vi "_Set PIC.vi"(1 "Count(uSec)":u8=20, 2 "Data":u32, 3 "Delay":u16) -> (0 "PIC Monitor":u32)   [LabVIEW 2018]
uses:
  <vilib>/eio/EIONode/EIONode.xnode
  <vilib>/rvi/DataTransferAndStorage/Container/XNode/niFpgaContainer.xnode
  <vilib>/rvi/eio/common/nirviEmuTemplateMethod_errors.vi
  <vilib>/rvi/Memory/Memory_Emulation/nirvimemoryFastEmulation.vi
  <vilib>/rvi/Memory/Memory_Emulation/nirvimemoryEmulation.vi
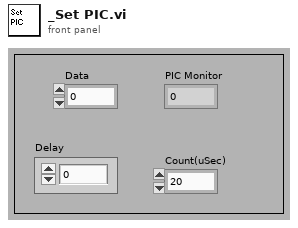
[diagram p1: front panel]
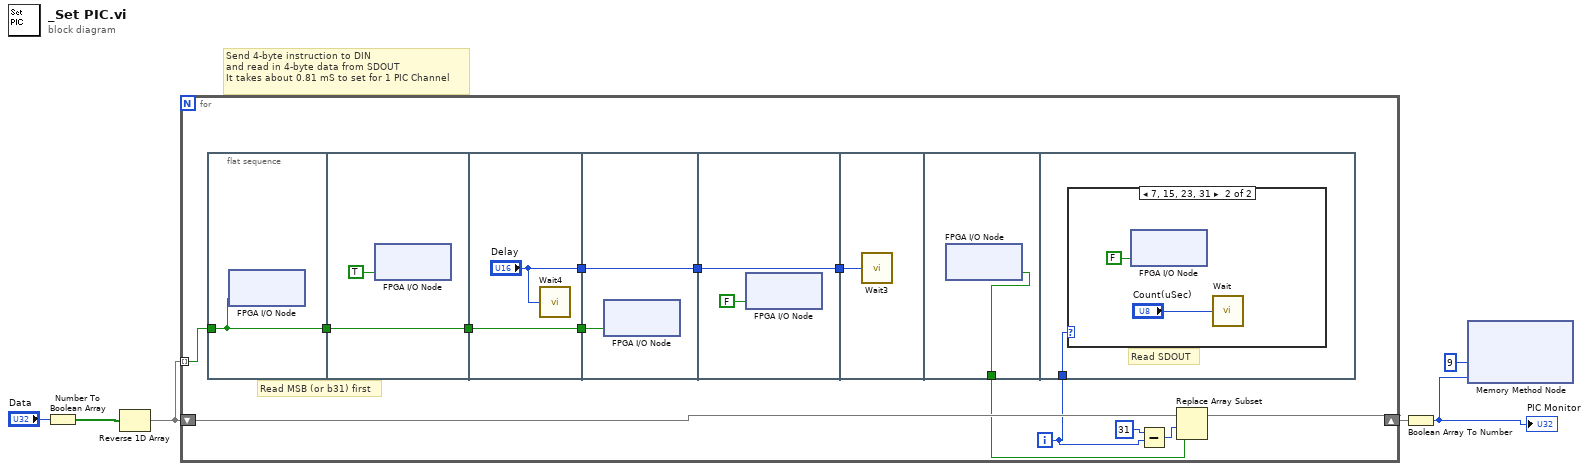
[diagram p0: block diagram]
diagram:
  # "Send 4-byte instruction to DIN\nand read in 4-byte data from SDOUT\nIt takes about 0.81 mS to set for 1 PIC Channel"
  n1 = Number To Boolean Array(number="Data") -> (Boolean array=w2:bool[])
  n2 = Reverse 1D Array(array=w2) -> (reversed array=w3:bool[])
  n3 = for {
    shift-right: [w18] -> w5
    shift-left: w3 -> [w19]
    tunnel: w3 -> [w15] mode=indexing
    i -> [w14]
    # "Read MSB (or b31) first"
    n4 = flat-sequence {
      tunnel: [w20] -> w11
      tunnel: w15 -> [w20]
      tunnel: w11 -> [w22]
      tunnel: [w22] -> w10
      tunnel: w10 -> [w24]
      tunnel: [w24] -> w13
      tunnel: ["Delay"] -> w12
      tunnel: w13 -> [w26]
      tunnel: [w25] -> w9
      tunnel: w12 -> [w25]
      tunnel: w9 -> [w28]
      tunnel: [w28] -> w8
      tunnel: w8 -> [w29]
      tunnel: [w30] -> w7
      tunnel: w14 -> [w31]
      frame #0 {
        n5 = xnode "FPGA I/O Node"("MOSI"=w20) -> ()  [unwired: 1 in, 1 out]
      }
      frame #1 {
        n6 = xnode "FPGA I/O Node"("SCLK"=TRUE) -> ()  [unwired: 1 in, 1 out]
      }
      frame #2 {
        n7 = call "Wait4"("Count(Ticks)"="Delay") -> ()  [unwired: 1 out]
      }
      frame #3 {
        n8 = xnode "FPGA I/O Node"("MOSI"=w26) -> ()  [unwired: 1 in, 1 out]
      }
      frame #4 {
        n9 = xnode "FPGA I/O Node"("SCLK"=FALSE) -> ()  [unwired: 1 in, 1 out]
      }
      frame #5 {
        n10 = call "Wait3"("Count(Ticks)"=w29) -> ()  [unwired: 1 out]
      }
      frame #6 {
        n11 = xnode "FPGA I/O Node"() -> ("MISO"=w30:bool)  [unwired: 1 in, 1 out]
      }
      frame #7 {
        # "Read SDOUT"
        n12 = case shown="7, 15, 23, 31" w31 {
          frame 0, Default {
          }
          frame 7, 15, 23, 31 {
            n13 = xnode "FPGA I/O Node"("MOSI"=FALSE) -> ()  [unwired: 1 in, 1 out]
            n14 = call "Wait"("Count(uSec)"="Count(uSec)") -> ()  [unwired: 1 out]
          }
        }
      }
    }
    n15 = Subtract(x=31, y=w14) -> (x-y=w16:i32)
    n16 = Replace Array Subset(array=w19, new element=w7, index=w16) -> (w18:bool[])
  }
  n17 = Boolean Array To Number(Boolean array=w5) -> (number=w1:u32)
  "PIC Monitor" <- w1
  n18 = xnode ("Memory Method Node")("Address"=u32 9, "Data"=w1) -> ()  [unwired: 1 in, 1 out]
